vi "SetTxLabelDecimation.vi"(6 "SectionBaseRate":i32, 7 "ScheduledSDI":bool, 8 "error in (no error)":errorcluster, 11 "Labels Settings In":T1[](array[typedef]) {"Words"."Param Setting"."Num Bits" min=1 max=32; "Words"."Param Setting"."Start Bit" min=8 max=31; "Words"."Block Data Refs"."Data Reference" format="%.0x"; "Label" format="%.0o"}) -> (0 "error out":errorcluster, 3 "Label Settings Out":T1[](array[typedef]) {"Words"."Param Setting"."Num Bits" min=1 max=32; "Words"."Param Setting"."Start Bit" min=8 max=31; "Words"."Block Data Refs"."Data Reference" format="%.0x"; "Label" format="%.0o"})   [LabVIEW 2011, in "AIT 429 Custom Device.lvlib"]
uses:
  AIT 429 Custom Device.lvlib
  RT Controls/RT Label Settings.ctl
  Controls and Global/Label.ctl
  Controls and Global/transferPeriod.ctl
  RT Controls/Driver Data.ctl
  RT Controls/RT Word Settings.ctl
  <vilib>/NI Veristand/Custom Device API/Block Data Reference.ctl
  <vilib>/NI Veristand/Custom Device API/Data Reference.ctl
  RT Controls/RT Param Setting.ctl
  Controls and Global/Start Bit.ctl
  Controls and Global/Number of Bits.ctl
  Controls and Global/TransferType.ctl
  <vilib>/NI Veristand/Custom Device API/Custom Device API.lvlib
  <instrlib>/AIT 429/AIT 429.lvlib
  <userlib>/ARINC-429/Owl429.lvlib
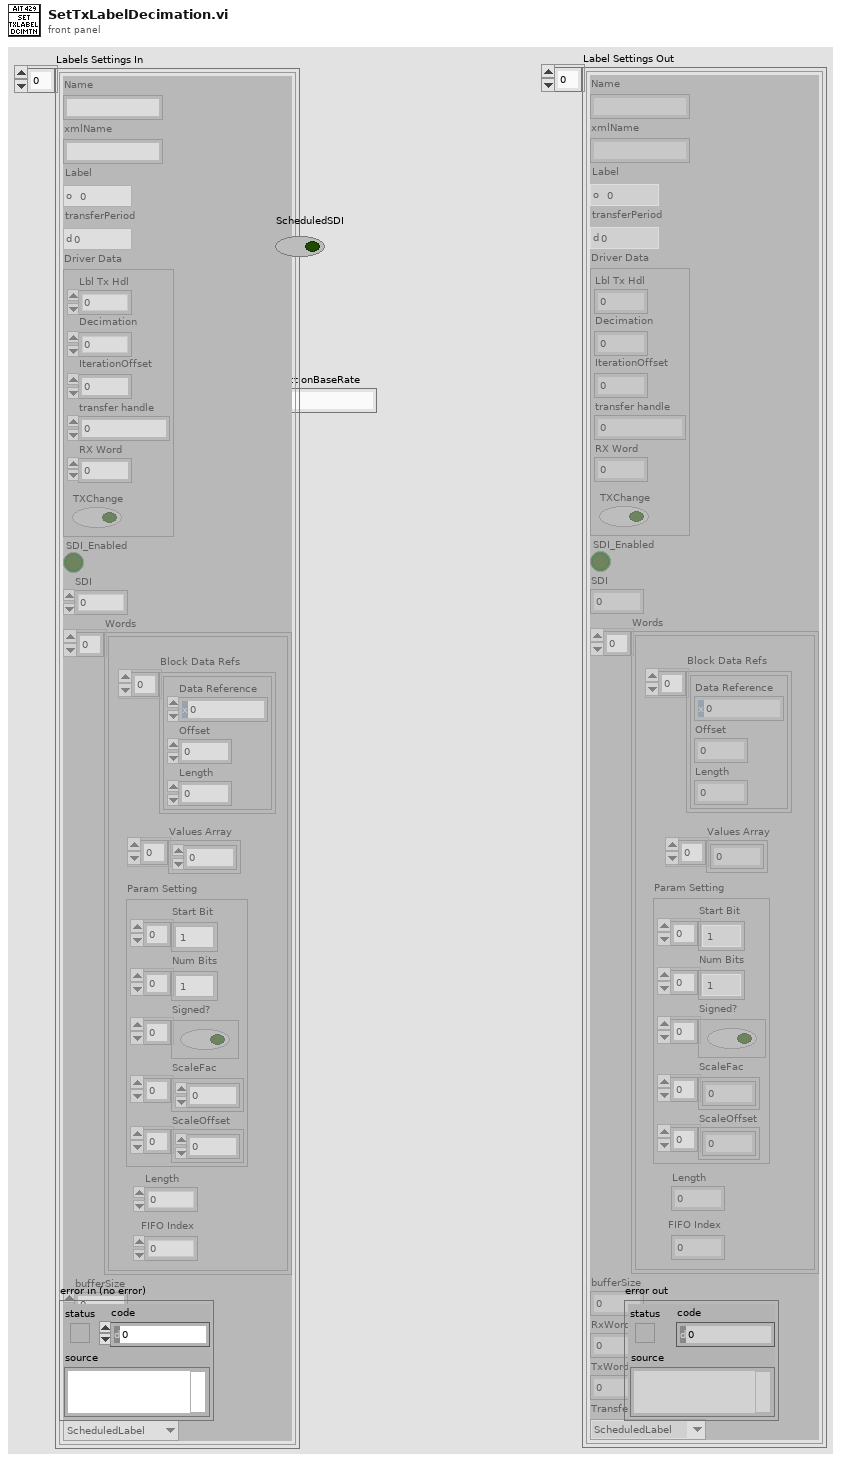
[diagram p1: front panel]
types:
  T1 = typedef "AIT 429 Custom Device.lvlib/RT Label Settings.ctl" = cluster{"Name":string, "xmlName":string, "Label":T2, "transferPeriod":T3, "Driver Data":T4, "SDI_Enabled":bool, "SDI":u8, "Words":T5[], "bufferSize":u32, "RxWordIdx":i32, "TxWordIdx":i32, "TransferType":T11}
  T2 = typedef "AIT 429 Custom Device.lvlib/Label.ctl" = u8
  T3 = typedef "AIT 429 Custom Device.lvlib/transferPeriod.ctl" = u32
  T4 = typedef "AIT 429 Custom Device.lvlib/Driver Data.ctl" = cluster{"Lbl Tx Hdl":u32, "Decimation":i32, "IterationOffset":i32, "transfer handle":u32, "RX Word":u32, "TXChange":bool}
  T5 = typedef "AIT 429 Custom Device.lvlib/RT Word Settings.ctl" = cluster{"Block Data Refs":T6[], "Values Array":dbl[], "Length":i32, "FIFO Index":i32, "Param Setting":T8}
  T6 = typedef "Custom Device API.lvlib/Block Data Reference.ctl" = cluster{"Data Reference":T7, "Offset":i32, "Length":i32}
  T7 = typedef "Custom Device API.lvlib/Data Reference.ctl" = i32
  T8 = typedef "AIT 429 Custom Device.lvlib/Rt Param Setting.ctl" = cluster{"Start Bit":T9[], "Num Bits":T10[], "Signed?":bool[], "ScaleFac":dbl[], "ScaleOffset":dbl[]}
  T9 = typedef "AIT 429 Custom Device.lvlib/Start Bit.ctl" = i32
  T10 = typedef "AIT 429 Custom Device.lvlib/Number of Bits.ctl" = i32
  T11 = typedef "AIT 429 Custom Device.lvlib/TransferType.ctl" = enum16{"ScheduledLabel", "Acyclic", "Block", "Strobe"}
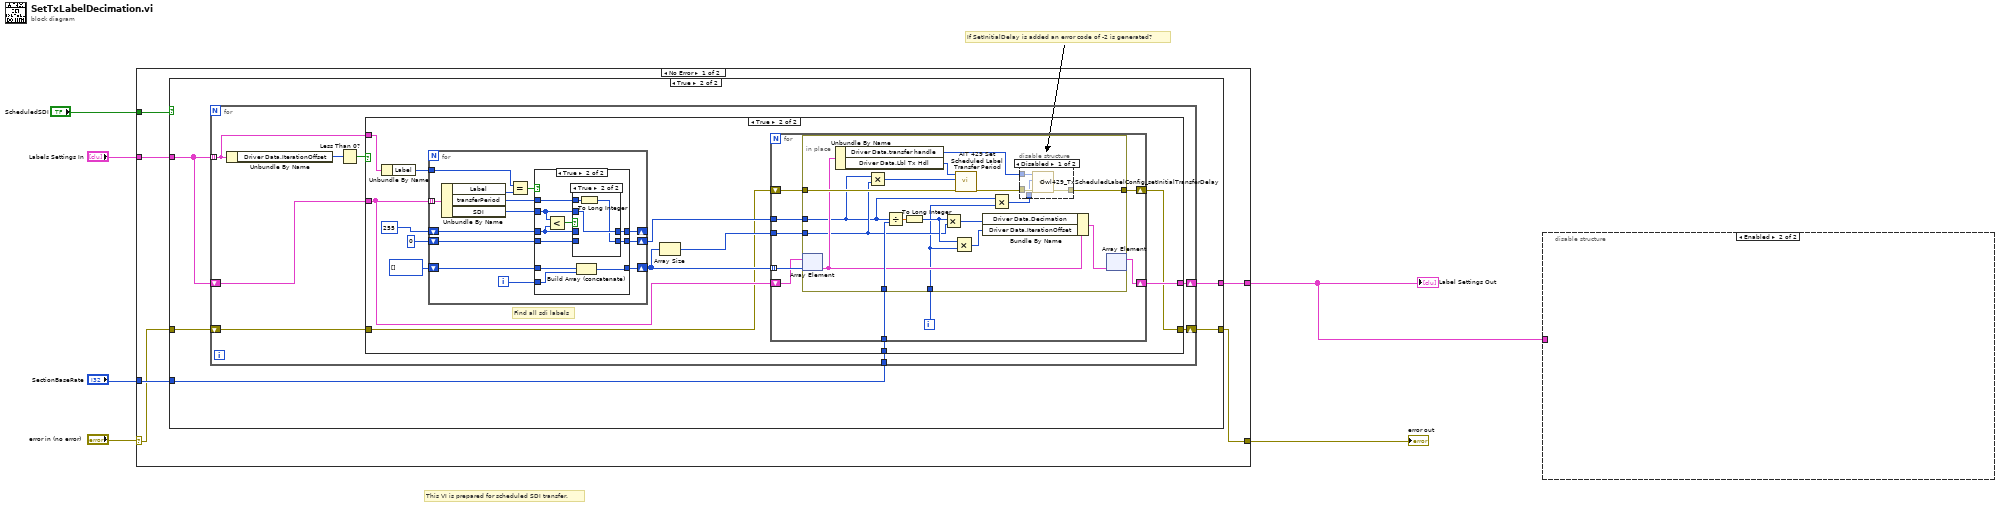
[diagram p0: block diagram]
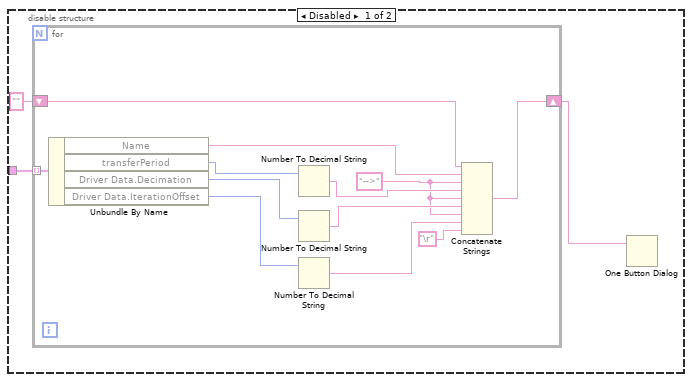
[diagram p2: hidden frame]
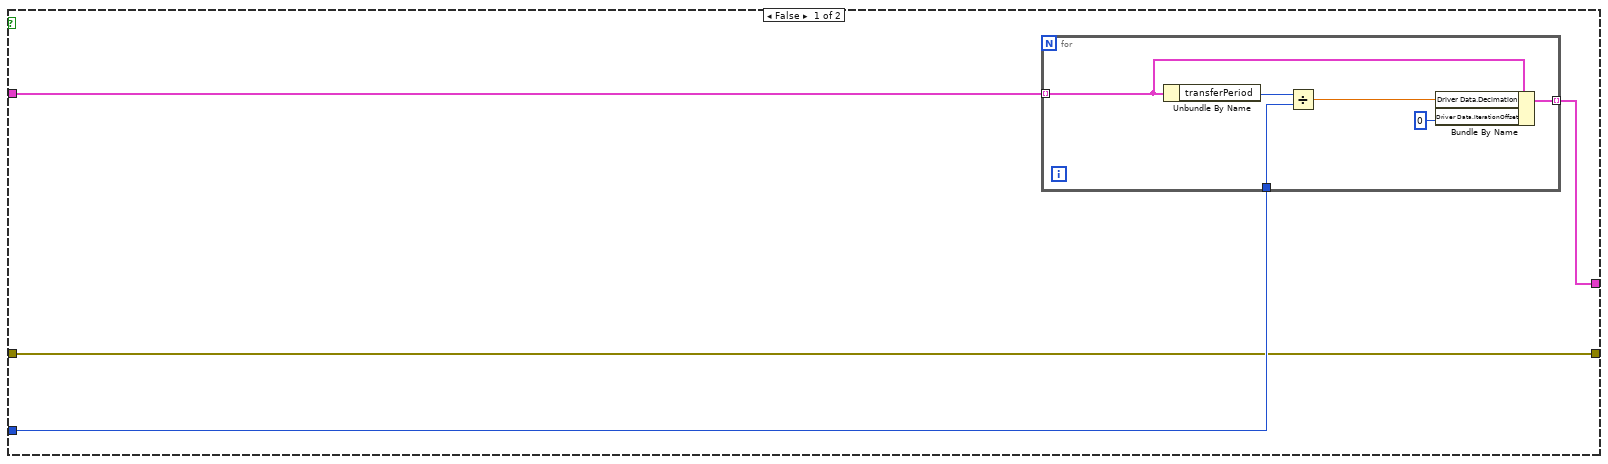
[diagram p3: hidden frame]
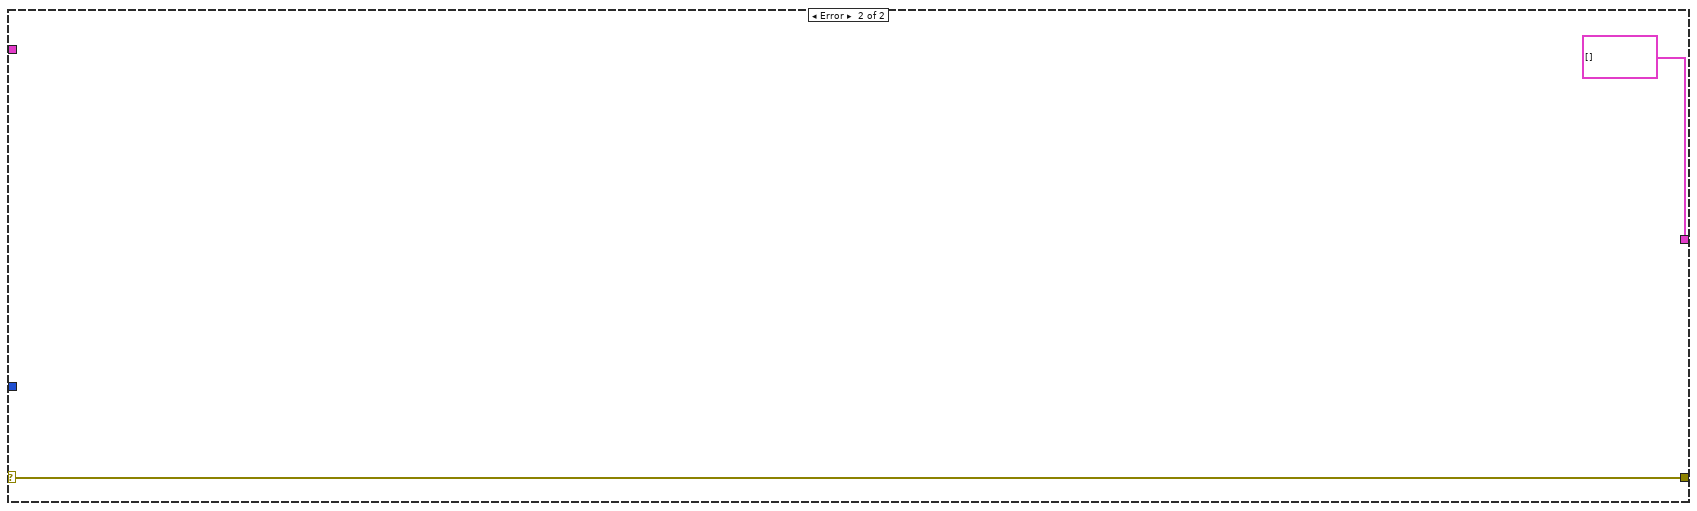
[diagram p8: hidden frame]
diagram:
  # "If SetInitialDelay is added an error code of -2 is generated?"
  # "This VI is prepared for scheduled SDI transfer."
  n1 = case shown="No Error" "error in (no error)" {
    selector: "error in (no error)" -> [w7 w113]
    tunnel: [w12 T1[] []] -> w1
    tunnel: "SectionBaseRate" -> [w11 _]
    tunnel: [w8 w113] -> w4
    tunnel: "Labels Settings In" -> [w10 _]
    tunnel: "ScheduledSDI" -> [w9 _]
    frame No Error {
      n2 = case shown="True" w9 {
        tunnel: [w16 w26] -> w12
        tunnel: w11 -> [w14 w23]
        tunnel: w10 -> [w15 w27]
        tunnel: [w13 w25] -> w8
        tunnel: w7 -> [w13 w24]
        frame False {
          n3 = for {
            tunnel: w15 -> [w20] mode=indexing
            tunnel: w14 -> [w21]
            tunnel: [w18] -> w16 mode=indexing
            n4 = Unbundle By Name(w20) -> ("transferPeriod"=w22:T3)
            n5 = Divide(x=w22, y=w21) -> (x/y=w19:dbl)
            n6 = Bundle By Name(cluster=w20, "Driver Data.Decimation"=w19, "Driver Data.IterationOffset"=0) -> (w18:T1)
          }
        }
        frame True {
          n7 = for {
            tunnel: w27 -> [w33] mode=indexing
            tunnel: w23 -> [w35]
            shift-right: [w30] -> w26
            shift-left: w27 -> [w34]
            shift-right: [w28] -> w25
            shift-left: w24 -> [w29]
            n8 = Unbundle By Name(w33) -> ("Driver Data.IterationOffset"=w32:i32)
            n9 = Less Than 0?(x=w32) -> (x < 0?=w31:bool)
            n10 = case shown="True" w31 {
              tunnel: w35 -> [_ w42]
              tunnel: w34 -> [w37 w44]
              tunnel: w33 -> [_ w50]
              tunnel: [w37 w41] -> w30
              tunnel: w29 -> [w36 w39]
              tunnel: [w36 w38] -> w28
              frame False {
              }
              frame True {
                # "Find all sdi labels"
                n11 = Unbundle By Name(w50) -> ("Label"=w49:T2)
                n12 = for {
                  shift-right: [w89] -> w45
                  shift-left: i32[] [] -> [w90]
                  tunnel: w44 -> [w94] mode=indexing
                  tunnel: w49 -> [w93]
                  shift-right: [w83] -> w43
                  shift-left: 0 -> [w85]
                  shift-right: [w82] -> _
                  shift-left: u8 255 -> [w84]
                  i -> [w88]
                  n13 = Unbundle By Name(w94) -> ("Label"=w92:T2, "transferPeriod"=w87:T3, "SDI"=w86:u8)
                  n14 = Equal?(x=w93, y=w92) -> (x = y?=w91:bool)
                  n15 = case shown="True" w91 {
                    tunnel: w90 -> [w97 w107]
                    tunnel: [w97 w105] -> w89
                    tunnel: w88 -> [_ w106]
                    tunnel: w87 -> [_ w102]
                    tunnel: w86 -> [_ w99]
                    tunnel: w85 -> [w95 w103]
                    tunnel: w84 -> [w96 w100]
                    tunnel: [w95 w101] -> w83
                    tunnel: [w96 w98] -> w82
                    frame False {
                    }
                    frame True {
                      n16 = Less?(x=w99, y=w100) -> (x < y?=w104:bool)
                      n17 = case shown="True" w104 {
                        tunnel: w103 -> [w108 _]
                        tunnel: w102 -> [_ w112]
                        tunnel: [w108 w110] -> w101
                        tunnel: w100 -> [w109 _]
                        tunnel: w99 -> [_ w111]
                        tunnel: [w109 w111] -> w98
                        frame False {
                        }
                        frame True {
                          n18 = To Long Integer(number=w112) -> (32bit integer=w110:i32)
                        }
                      }
                      n19 = Build Array (concatenate)(w107, w106) -> (w105:i32[])
                    }
                  }
                }
                n20 = Array Size(array=w45) -> (size(s)=w40:i32)
                n21 = for {
                  tunnel: w45 -> [w59] mode=indexing
                  tunnel: w40 -> [w53]
                  tunnel: w43 -> [w56]
                  tunnel: w42 -> [w55]
                  shift-right: [w57] -> w41
                  shift-left: w44 -> [w58]
                  shift-right: [w51] -> w38
                  shift-left: w39 -> [w52]
                  i -> [w54]
                  n22 = in-place {
                    in-place-border: w56 -> [w64]
                    in-place-border: w55 -> [w75]
                    in-place-border: w54 -> [w62]
                    in-place-border: w53 -> [w66]
                    in-place-border: w52 -> [w70]
                    in-place-border: [w68] -> w51
                    n23 = in-place-array #1(w58, w59) -> (w67:T1)
                    n24 = Unbundle By Name(w67) -> ("Driver Data.transfer handle"=w60:u32, "Driver Data.Lbl Tx Hdl"=w61:u32)
                    n25 = Multiply(x=w64, y=w66) -> (x*y=w65:i32)
                    n26 = Divide(x=w64, y=w75) -> (x/y=w72:dbl)
                    n27 = To Long Integer(number=w72) -> (32bit integer=w71:i32)
                    n28 = Multiply(x=w71, y=w66) -> (x*y=w73:i32)
                    n29 = Multiply(x=w71, y=w62) -> (x*y=w74:i32)
                    n30 = call <instrlib>:"AIT 429 Set Scheduled Label Transfer Period.vi"("error in (no error)"=w70, "transfer period"=w65, "scheduled label handle"=w61) -> ("error out"=w69:errorcluster)  [unwired: 7 in, 1 out]
                    n31 = Bundle By Name(cluster=w67, "Driver Data.Decimation"=w73, "Driver Data.IterationOffset"=w74) -> (w76:T1)
                    n32 = Multiply(x=w64, y=w62) -> (x*y=w63:i32)
                    n33 = disable-structure shown="Disabled" {
                      disable-tunnel: w69 -> [w80 w81]
                      disable-tunnel: [w79 w81] -> w68
                      disable-tunnel: w63 -> [w78 _]
                      disable-tunnel: w60 -> [w77 _]
                      frame Disabled {
                        n34 = call <userlib>:"Owl429_TxScheduledLabelConfig_setInitialTransferDelay.vi"("error in (no error)"=w80, "delay"=w78, "label config handle"=w77) -> ("error out"=w79:errorcluster)  [unwired: 7 in, 1 out]
                      }
                      frame Enabled {
                      }
                    }
                    n35 = in-place-array #1(w76) -> (w57:T1[])  [unwired: 1 out]
                  }
                }
              }
            }
          }
        }
      }
    }
    frame Error {
    }
  }
  "Label Settings Out" <- w1
  "error out" <- w4
  n36 = disable-structure shown="Enabled" {
    disable-tunnel: w1 -> [w117 _]
    frame Disabled {
      n37 = for {
        tunnel: w117 -> [w129] mode=indexing
        shift-right: [w120] -> w115
        shift-left: "" -> [w118]
        w122 = "-->" ("string")
        n38 = Unbundle By Name(w129) -> ("Name"=w125:string, "transferPeriod"=w128:T3, "Driver Data.Decimation"=w127:i32, "Driver Data.IterationOffset"=w126:i32)
        n39 = Number To Decimal String(number=w128) -> (decimal integer string=w124:string)  [unwired: 1 in]
        n40 = Number To Decimal String(number=w127) -> (decimal integer string=w123:string)  [unwired: 1 in]
        n41 = Number To Decimal String(number=w126) -> (decimal integer string=w121:string)  [unwired: 1 in]
        n42 = Concatenate Strings(w118, w125, w122, w124, w122, w123, w122, w121, "\r") -> (w120:string)
      }
      n43 = One Button Dialog(message=w115) -> ()  [unwired: 1 in, 1 out]
    }
    frame Enabled {
    }
  }
